vi "198 Motor Init.vi"(1 "error in":errorcluster) -> (0 "error out":errorcluster)   [LabVIEW 2014]
uses:
  <vilib>/Rock Robotics/SystemInterfaces/DIO/FPGA_DIOPWMChannel.ctl
  <vilib>/Rock Robotics/WPI/SafetyOutput/WPI_SafetyOutputConfigMenu.ctl
  <vilib>/Rock Robotics/WPI/MotorControl/WPI_MotorControlOpen Victor.vi
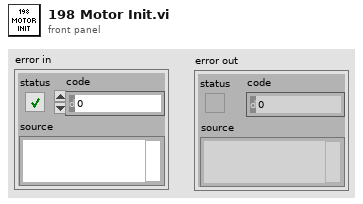
[diagram p1: front panel]
types:
  T1 = typedef "WPI_SafetyOutputConfigMenu.ctl" = enum16{"Enable", "Disable"}
  T2 = typedef "FPGA_DIOPWMChannel.ctl" = enum8{"PWM 0", "PWM 1", "PWM 2", "PWM 3", "PWM 4", "PWM 5", "PWM 6", "PWM 7", "PWM 8", "PWM 9", "PWM MXP 0", "PWM MXP 1", "PWM MXP 2", "PWM MXP 3", "PWM MXP 4", "PWM MXP 5", "PWM MXP 6", "PWM MXP 7", "PWM MXP 8", "PWM MXP 9", "Invalid"}
  T3 = typedef "WPI_MotorControlDeviceRef.ctl" = cluster{"DeviceStatus":errorcluster, "Type":T4, "PWM":cluster{"Controller":T5, "PWM Channel":T2, "DeadBand":T6}, "CAN":cluster{"Device Number":u8, "Control Mode":T7, "Semaphore":T8, "Max Vout":dbl, "TalonSRX Control Mode":T9}, "Invert":bool, "TransformRef":T10, "InvTransformRef":T10}
  T4 = typedef "WPI_MotorControlType.ctl" = enum16{"PWM", "CAN", "CANTalonSRX"}
  T5 = typedef "FPGA_TypedefDigitalModule.ctl" = enum16{"Controller 1"}
  T6 = typedef "WPI_PWMDeadband.ctl" = cluster{"Name":string, "maxPositivePwm":i32, "minPositivePwm":i32, "centerPwm":i32, "maxNegativePwm":i32, "minNegativePwm":i32, "angularRange":u16}
  T7 = typedef "WPI_CANJaguar_ControlMode.ctl" = enum8{"Percent VBus", "Current", "Speed", "Position", "Voltage"}
  T8 = typedef "Semaphore RefNum" = refnum<k1>
  T9 = typedef "WPI_CANTalonSRX_APIControlMode.ctl" = enum8{"Percent VBus", "Speed", "Position", "Slave", "Unchanged / Invalid"}
  T10 = typedef "WPI_PWMTransform_ConPane.ctl" = refnum<vi>
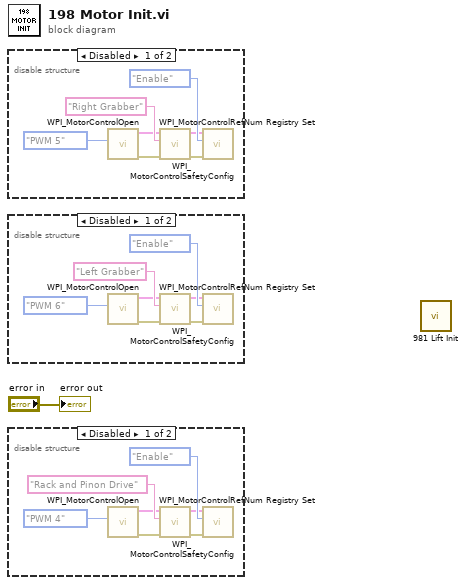
[diagram p0: block diagram]
diagram:
  n1 = disable-structure shown="Disabled" {
    frame Disabled {
      n2 = call-poly <vilib>:"WPI_MotorControlOpen.vi"("PWM Channel"=FPGA_DIOPWMChannel."PWM 5") -> ("error out"=w7:errorcluster, "MotorControlDeviceRef"=w3:T3)  [unwired: 9 in]
      n3 = call <vilib>:"WPI_MotorControlRefNum Registry Set.vi"("error in (no error)"=w7, "refnum name"="Right Grabber", "MotorControlDevRef"=w3) -> ("error out"=w6:errorcluster, "MotorControlDevRef"=w5:T3)  [unwired: 7 in]
      n4 = call <vilib>:"WPI_MotorControlSafetyConfig.vi"("error in (no error)"=w6, "mode"=WPI_SafetyOutputConfigMenu."Enable", "MotorControlDevRef"=w5) -> ()  [unwired: 7 in, 2 out]
    }
    frame Enabled {
    }
  }
  n5 = disable-structure shown="Disabled" {
    frame Disabled {
      n6 = call-poly <vilib>:"WPI_MotorControlOpen.vi"("PWM Channel"=FPGA_DIOPWMChannel."PWM 6") -> ("error out"=w14:errorcluster, "MotorControlDeviceRef"=w10:T3)  [unwired: 9 in]
      n7 = call <vilib>:"WPI_MotorControlRefNum Registry Set.vi"("error in (no error)"=w14, "refnum name"="Left Grabber", "MotorControlDevRef"=w10) -> ("error out"=w13:errorcluster, "MotorControlDevRef"=w12:T3)  [unwired: 7 in]
      n8 = call <vilib>:"WPI_MotorControlSafetyConfig.vi"("error in (no error)"=w13, "mode"=WPI_SafetyOutputConfigMenu."Enable", "MotorControlDevRef"=w12) -> ()  [unwired: 7 in, 2 out]
    }
    frame Enabled {
    }
  }
  n9 = disable-structure shown="Disabled" {
    frame Disabled {
      n10 = call-poly <vilib>:"WPI_MotorControlOpen.vi"("PWM Channel"=FPGA_DIOPWMChannel."PWM 4") -> ("error out"=w21:errorcluster, "MotorControlDeviceRef"=w17:T3)  [unwired: 9 in]
      n11 = call <vilib>:"WPI_MotorControlRefNum Registry Set.vi"("error in (no error)"=w21, "refnum name"="Rack and Pinon Drive", "MotorControlDevRef"=w17) -> ("error out"=w20:errorcluster, "MotorControlDevRef"=w19:T3)  [unwired: 7 in]
      n12 = call <vilib>:"WPI_MotorControlSafetyConfig.vi"("error in (no error)"=w20, "mode"=WPI_SafetyOutputConfigMenu."Enable", "MotorControlDevRef"=w19) -> ()  [unwired: 7 in, 2 out]
    }
    frame Enabled {
    }
  }
  n13 = call "981 Lift Init.vi"() -> ()  [unwired: 1 in, 1 out]
  "error out" <- "error in"
